vi "Disconnect.vi"(8 "Error In":errorcluster, 11 "Agent In":refnum<class "Agent.lvclass">) -> (0 "Error Out":errorcluster, 3 "Agent Out":refnum<class "Agent.lvclass">)   [LabVIEW 2021, in "Field_RnD_Services_LIBSSH2_Toolkit.lvlib" / "Agent.lvclass"]
doc: "Disconnects and closes the connection to the SSH-agent application. This should be called before the Agent object is destroyed."
uses:
  220524-VNA RP FLAT.llb/Agent.lvclass
  220524-VNA RP FLAT.llb/Agent.lvclass/Agent.ctl
  220524-VNA RP FLAT.llb/Field_RnD_Services_LIBSSH2_Toolkit.lvlib
  220524-VNA RP FLAT.llb/Session.lvclass
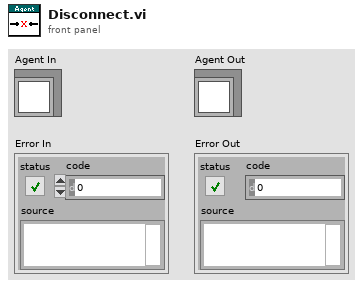
[diagram p1: front panel]
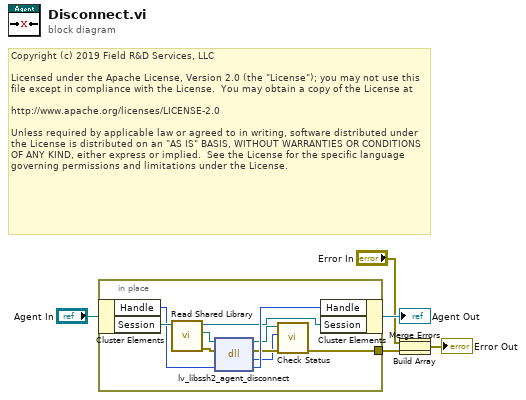
[diagram p0: block diagram]
diagram:
  # "Copyright (c) 2019 Field R&D Services, LLC\n\nLicensed under the Apache License, Version 2.0 (the \"License\"); you may not use this file except in compliance with the License.  You may obtain a copy of the License at\n\nhttp://www.apache.org/licenses/LICENSE-2.0\n\nUnless required by applicable law or agreed to in writing, software distributed under the License is distributed on an \"AS IS\" BASIS, WITHOUT WARRANTIES OR CONDITIONS OF ANY KIND, either express or implied.  See the License for the specific language governing permissions and limitations under the License."
  n1 = in-place {
    in-place-border: [w13] -> w6
    n2 = in-place-cluster #1("Agent In") -> ("Handle"=w8:u64, "Session"=w11:refnum<class "Session.lvclass">)
    n3 = call "Read Shared Library.vi"("Session In"=w11) -> ("Erorr Out"=w9:errorcluster, "libssh2lv Shared Library"=w10:path, "Session Out"=w7:refnum<class "Session.lvclass">)  [unwired: 8 in]
    n4 = dll-call lib="libssh2lv.*" fn="lv_libssh2_agent_disconnect"(path in=w10, error in=w9, "handle"=w8) -> (path out=w14:path, error out=w15:errorcluster, "result"=w12:i32, "handle"=w16:u64)  [unwired: 1 in]
    n5 = call "Check Status.vi"("Error In"=w15, "Status"=w12, "libssh2lv Shared Library In"=w14) -> ("Error Out"=w13:errorcluster)  [unwired: 7 in, 1 out]
    n6 = in-place-cluster #1("Handle"=w16, "Session"=w7) -> (→"Agent Out":refnum<class "Agent.lvclass">)
  }
  n7 = Build Array("Error In", w6) -> (w1:errorcluster[])
  n8 = Merge Errors(w1) -> (→"Error Out":errorcluster)
